vi "TR_MouseStatus.vi"(11 "Mouse in":refnum<class "Mouse.lvclass">) -> ()   [LabVIEW 2021, in "InputDevice.lvlib" / "Mouse.lvclass"]
uses:
  Mouse.lvclass
  eb7bb245-cb1a-4027-9ed5-b4438251725f.vi
  8ae88d8c-86e8-4183-9e02-5cb064982b42.vi
  <vilib>/Utility/inputDevices.llb/mouseAcquire.vi
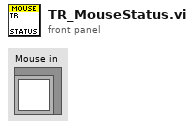
[diagram p1: front panel]
types:
  T1 = typedef "Mouse.lvclass/data.ctl" = cluster{"DeviceID":refnum<k1>, "MouseButtonInfo":refnum<user-event>, "MouseAxisInfo":refnum<user-event>, "MouseInfoEvents":refnum<event-registration>, "StopNotifier":refnum<notifier>}
  T2 = cluster{"Horizontal":i32, "Vertical":i32, "Scrolling":i32}
  T3 = cluster{"button 1":bool, "button 2":bool, "button 3":bool, "button 4":bool}
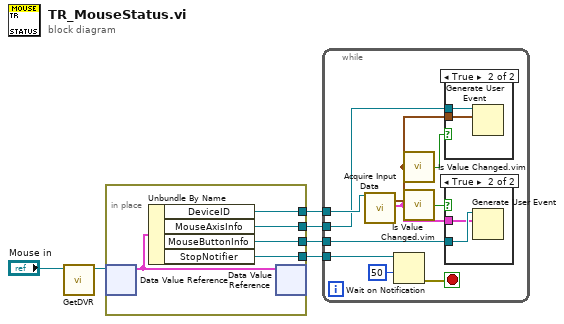
[diagram p0: block diagram]
diagram:
  n1 = call "GetDVR.vi"("Mouse"="Mouse in") -> ("DVR"=w5:refnum<data-value>)  [unwired: 9 in, 1 out]
  n2 = in-place {
    in-place-border: [w11] -> w4
    in-place-border: [w10] -> w3
    in-place-border: [w9] -> w2
    in-place-border: [w8] -> w1
    n3 = in-place-dvr #1(w5) -> (w7:T1)  [unwired: 1 out]
    n4 = Unbundle By Name(w7) -> ("DeviceID"=w11:refnum<k1>, "MouseAxisInfo"=w10:refnum<user-event>, "MouseButtonInfo"=w9:refnum<user-event>, "StopNotifier"=w8:refnum<notifier>)
    n5 = in-place-dvr #1(w7) -> ()  [unwired: 2 out]
  }
  n6 = while {
    tunnel: w4 -> [w21]
    tunnel: w3 -> [w19]
    tunnel: w2 -> [w15]
    tunnel: w1 -> [w13]
    stop <- w14 stop-if-true
    n7 = call-poly <vilib>:"Acquire Input Data.vi"("device ID"=w21) -> ("axis info"=w18:T2, "button info"=w16:T3)  [unwired: 15 in, 2 out]
    n8 = Wait on Notification(notifier=w13, timeout in ms (-1)=50) -> (error out=w14:errorcluster)  [unwired: 2 in, 3 out]
    n9 = call "Is Value Changed.vim"("value"=w18) -> ("changed or first call?"=w20:bool)
    n10 = call "Is Value Changed.vim"("value"=w16) -> ("changed or first call?"=w17:bool)
    n11 = case shown="True" w20 {
      tunnel: w19 -> [_ w25]
      tunnel: w18 -> [_ w24]
      frame False {
      }
      frame True {
        n12 = Generate User Event(user event=w25, event data cluster=w24) -> ()  [unwired: 2 in, 2 out]
      }
    }
    n13 = case shown="True" w17 {
      tunnel: w15 -> [_ w23]
      tunnel: w16 -> [_ w22]
      frame False {
      }
      frame True {
        n14 = Generate User Event(user event=w23, event data cluster=w22) -> ()  [unwired: 2 in, 2 out]
      }
    }
  }
